vi "Camera Setup IA.vi"(8 "error in (no error)":errorcluster, 10 "Camera Setup":cluster{"Exposure Time":i32}, 11 "Image Acquisition in":refnum<class "Image Acquisition.lvclass">) -> (0 "error out":errorcluster, 3 "Image Acquisition out":refnum<class "Image Acquisition.lvclass">)   [LabVIEW 2019, in "Image Acquisition.lvlib" / "Image Acquisition.lvclass"]
uses:
  Image Acquisition.lvclass
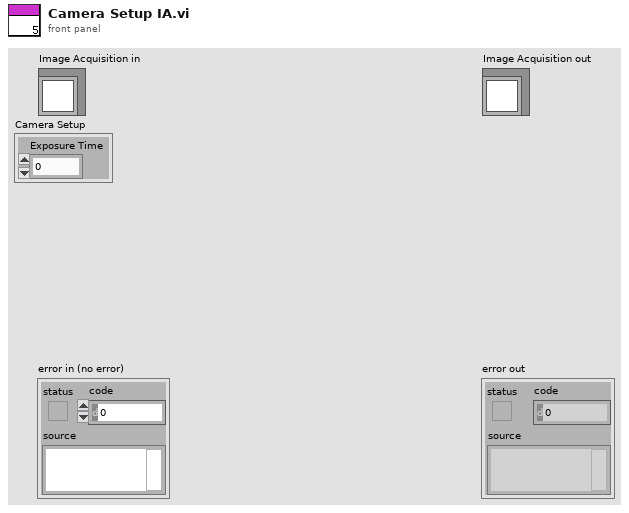
[diagram p1: front panel]
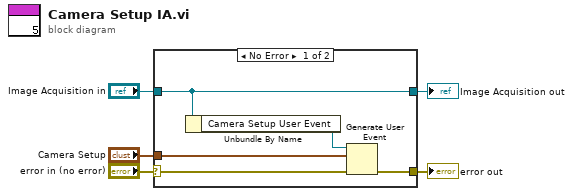
[diagram p0: block diagram]
diagram:
  n1 = case shown="No Error" "error in (no error)" {
    selector: "error in (no error)" -> [w7 w12]
    tunnel: [w6 w12] -> w4
    tunnel: [w10 w11] -> w2
    tunnel: "Image Acquisition in" -> [w10 w11]
    tunnel: "Camera Setup" -> [w8 _]
    frame No Error {
      n2 = Unbundle By Name(w10) -> ("Camera Setup User Event"=w9:refnum<user-event>)
      n3 = Generate User Event(user event=w9, event data cluster=w8, error in=w7) -> (error out=w6:errorcluster)  [unwired: 1 in, 1 out]
    }
    frame Error {
    }
  }
  "error out" <- w4
  "Image Acquisition out" <- w2
